vi "V3 - Copy to import to main.vi"() -> ()   [LabVIEW 2024]
uses:
  <vilib>/Utility/file.llb/Read Delimited Spreadsheet (string).vi
  <vilib>/Utility/file.llb/Write Delimited Spreadsheet (string).vi
panel:
  out "Array 3":string[](array[string])
  out "Path":path=path "C:/Users/willi/GITHUB/TG/OBJ 2 - RECOLECCION DE DATOS/registro-usuarios.csv"
  out "ActualUser":i32
  out "Array 2":i32[](array[numeric])
  out "Array":T1(array[cluster])
  in  "Tab Control":enum32{"Seleccionar ", "Registrar"}(tab)
  in  "Combo Box":string(combo)
  in  "Registrar Usuario":T2 {"Edad" format="%#_13g"}
  in  "registrButt":bool
  in  "stop":bool
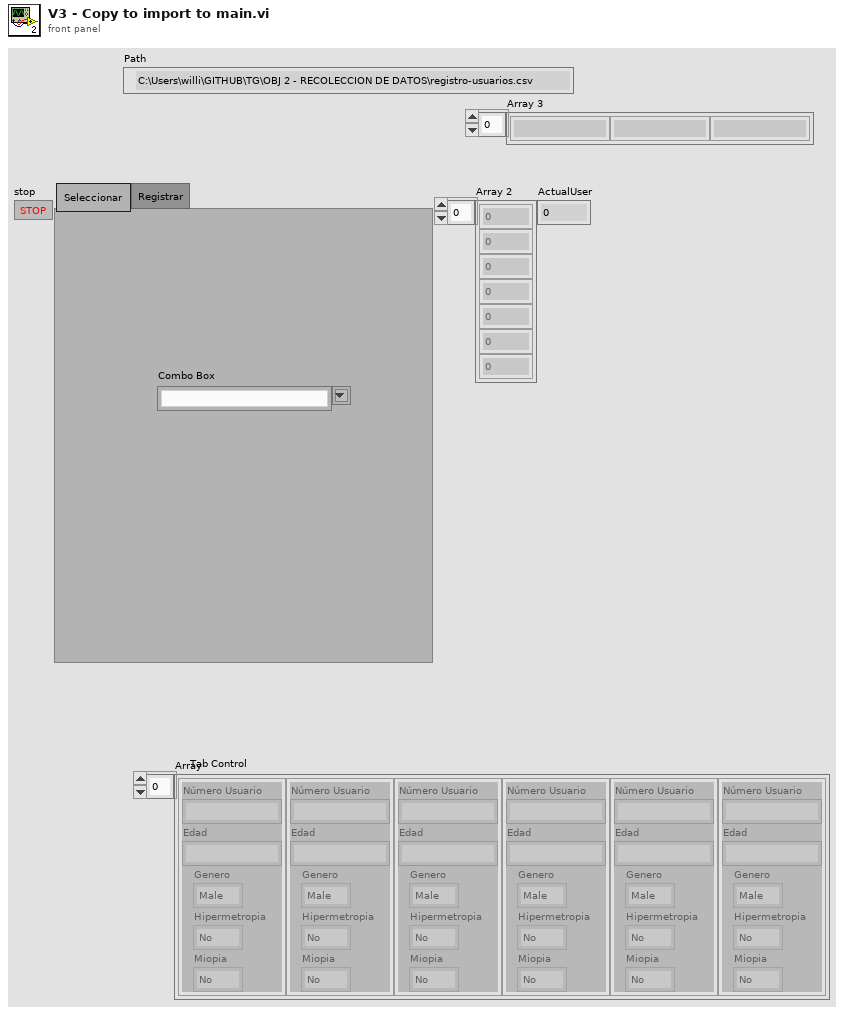
[diagram p1: front panel]
types:
  T1 = cluster{"Número Usuario":string, "Edad":string, "Genero":enum16{"Male", "Female"}, "Hipermetropia":enum16{"No", "Si"}, "Miopia":enum16{"No", "Si"}}[]
  T2 = cluster{"Genero":enum16{"Male", "Female"}, "Edad":dbl, "Hipermetropia":enum16{"No", "Si"}, "Miopia":enum16{"No", "Si"}}
  T3 = cluster{"Número Usuario":string, "Edad":string, "Genero":enum16{"Male", "Female"}, "Hipermetropia":enum16{"No", "Si"}, "Miopia":enum16{"No", "Si"}}
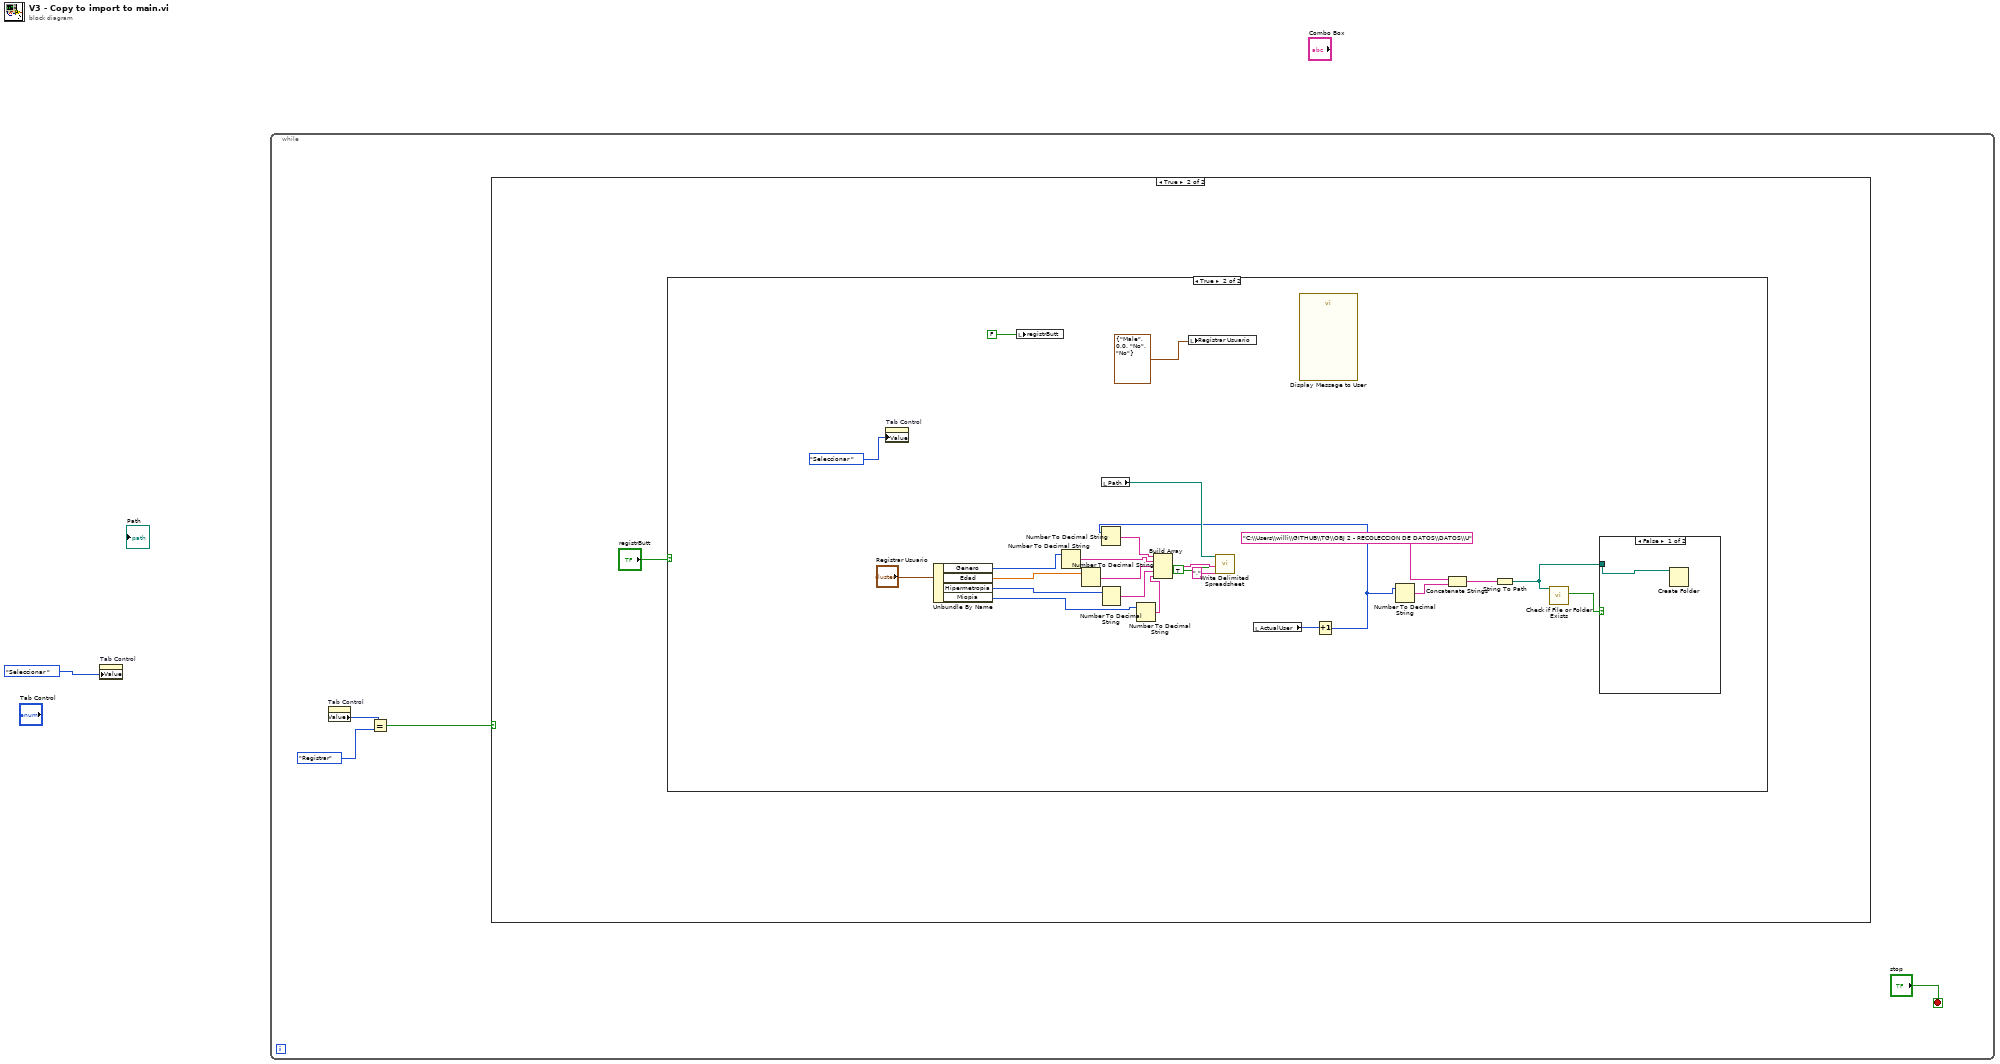
[diagram p0: block diagram]
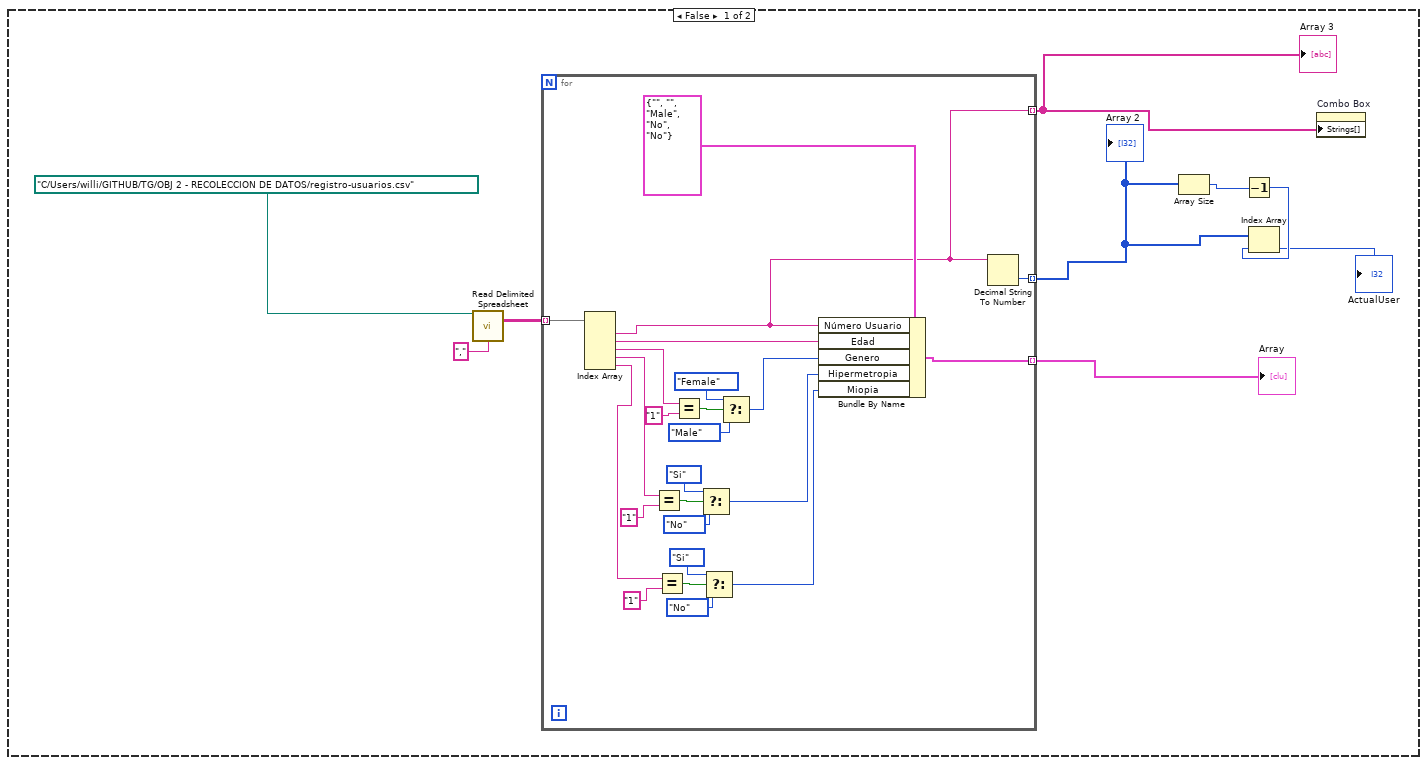
[diagram p2: hidden frame]
diagram:
  n1 = property on="Tab Control" class="TabCtl (strict)"("Value"=enum32{"Seleccionar ", "Registrar"}."Seleccionar " ("Tab Control")) -> ()  [unwired: 2 in, 2 out]
  n2 = while {
    stop <- "stop" stop-if-true
    n3 = property on="Tab Control" class="TabCtl (strict)"() -> ("Value"=w4:enum32{"Seleccionar ", "Registrar"})  [unwired: 2 in, 2 out]
    n4 = Equal?(x=w4, y=enum32{"Seleccionar ", "Registrar"}."Registrar" ("Tab Control")) -> (x = y?=w2:bool)
    n5 = case shown="True" w2 {
      frame False {
        n6 = call-poly <vilib>:"Read Delimited Spreadsheet.vi"("file path (dialog if empty)"=path "C:/Users/willi/GITHUB/TG/OBJ 2 - RECOLECCION DE DATOS/registro-usuarios.csv", "delimiter (\\t)"="," ("delimiter (\\t)")) -> ("all rows"=w13:string[][])  [unwired: 8 in, 5 out]
        n7 = for {
          tunnel: w13 -> [w38] mode=indexing
          tunnel: [w17] -> w12 mode=indexing
          tunnel: [w16] -> w10 mode=indexing
          tunnel: [w15] -> w6 mode=indexing
          n8 = Index Array(array=w38) -> (element #1=w15:string, element #2=w36:string, element #3=w34:string, element #4=w25:string, element #5=w19:string)  [unwired: 5 in]
          n9 = Equal?(x=w25, y="1") -> (x = y?=w28:bool)
          n10 = Equal?(x=w19, y="1") -> (x = y?=w22:bool)
          n11 = Equal?(x=w34, y="1") -> (x = y?=w33:bool)
          n12 = Select(t=enum16{"No", "Si"}."Si" ("Hipermetropia"), s=w28, f=enum16{"No", "Si"}."No" ("Hipermetropia")) -> (s? t:f=w24:enum16{"No", "Si"})
          n13 = Select(t=enum16{"No", "Si"}."Si" ("Hipermetropia"), s=w22, f=enum16{"No", "Si"}."No" ("Hipermetropia")) -> (s? t:f=w18:enum16{"No", "Si"})
          n14 = Select(t=enum16{"Male", "Female"}."Female" ("Genero"), s=w33, f=enum16{"Male", "Female"}."Male" ("Genero")) -> (s? t:f=w30:enum16{"Male", "Female"})
          n15 = Bundle By Name(cluster=T3 {"Número Usuario"="", "Edad"="", "Genero"=enum."Male", "Hipermetropia"=enum."No", "Miopia"=enum."No"} ("Registrar Usuario"), "Número Usuario"=w15, "Edad"=w36, "Genero"=w30, "Hipermetropia"=w24, "Miopia"=w18) -> (w17:T3)
          n16 = Decimal String To Number(string=w15) -> (number=w16:i32)  [unwired: 2 in, 1 out]
        }
        "Array" <- w12
        "Array 2" <- w10
        "Array 3" <- w6
        n17 = Array Size(array=w10) -> (size(s)=w9:i32)
        n18 = Decrement(x=w9) -> (x-1=w8:i32)
        n19 = Index Array(array=w10, index=w8) -> (element=→"ActualUser":i32)
        n20 = property on="Combo Box" class="CmbBox"("Strings[]"=w6) -> ()  [unwired: 2 in, 2 out]
      }
      frame True {
        n21 = case shown="True" "registrButt" {
          frame False {
          }
          frame True {
            n22 = property on="Tab Control" class="TabCtl (strict)"("Value"=enum32{"Seleccionar ", "Registrar"}."Seleccionar " ("Tab Control")) -> ()  [unwired: 2 in, 2 out]
            n23 = Unbundle By Name("Registrar Usuario") -> ("Genero"=w53:enum16{"Male", "Female"}, "Edad"=w52:dbl, "Hipermetropia"=w51:enum16{"No", "Si"}, "Miopia"=w50:enum16{"No", "Si"})
            n24 = local write "registrButt"(FALSE) -> ()
            n25 = Number To Decimal String(number=w53) -> (decimal integer string=w54:string)  [unwired: 1 in]
            n26 = Number To Decimal String(number=w52) -> (decimal integer string=w57:string)  [unwired: 1 in]
            n27 = local read "Path"() -> (w46:path)
            n28 = Number To Decimal String(number=w51) -> (decimal integer string=w58:string)  [unwired: 1 in]
            n29 = Number To Decimal String(number=w50) -> (decimal integer string=w59:string)  [unwired: 1 in]
            n30 = local write "Registrar Usuario"(T2 {"Genero"=enum."Male", "Edad"=0.0, "Hipermetropia"=enum."No", "Miopia"=enum."No"} ("Registrar Usuario")) -> ()
            n31 = local read "ActualUser"() -> (w41:i32)
            n32 = call "Display Message to User"() -> ()  [unwired: 10 in, 2 out]
            n33 = Increment(x=w41) -> (x+1=w40:i32)
            n34 = Number To Decimal String(number=w40) -> (decimal integer string=w49:string)  [unwired: 1 in]
            n35 = Build Array(w49, w54, w57, w58, w59) -> (w62:string[])
            n36 = call-poly <vilib>:"Write Delimited Spreadsheet.vi"("file path (dialog if empty)"=w46, "1D data"=w62, "append to file? (new file:F)"=TRUE, "delimiter (\\t)"="," ("delimiter (\\t)")) -> ()  [unwired: 10 in, 2 out]
            n37 = Number To Decimal String(number=w40) -> (decimal integer string=w48:string)  [unwired: 1 in]
            n38 = Concatenate Strings("C:\\Users\\willi\\GITHUB\\TG\\OBJ 2 - RECOLECCION DE DATOS\\DATOS\\U" ("string"), w48) -> (w45:string)
            n39 = String To Path(string=w45) -> (path=w43:path)
            n40 = call <vilib>:"Check if File or Folder Exists.vi"("path"=w43) -> ("file or folder exists?"=w44:bool)  [unwired: 8 in, 2 out]
            n41 = case shown="False" w44 {
              tunnel: w43 -> [w64 _]
              frame False {
                n42 = Create Folder(path (use dialog)=w64) -> ()  [unwired: 2 in, 3 out]
              }
              frame True {
              }
            }
          }
        }
      }
    }
  }
